vi "F Dwf Analog Impedance Amplitude Get.vi"(8 "error in (no error)":errorcluster, 10 "pvolts":dbl, 11 "hdwf":i32) -> (0 "error out":errorcluster, 2 "pvolts out":dbl, 3 "function return":i32)   [LabVIEW 2019, in "Olasdwf.lvlib"]
doc: "DWFAPI int FDwfAnalogImpedanceAmplitudeGet(HDWF hdwf, double *pvolts);"
uses:
  Olasdwf.lvlib
  Windows/System32/dwf.dll
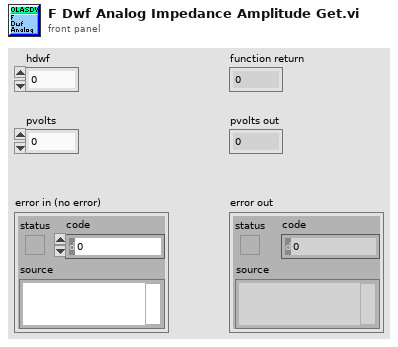
[diagram p1: front panel]
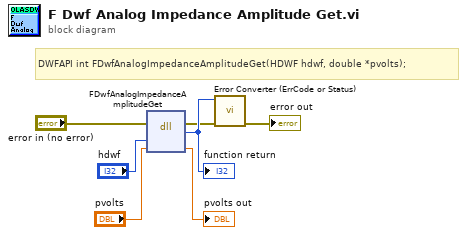
[diagram p0: block diagram]
diagram:
  # "DWFAPI int FDwfAnalogImpedanceAmplitudeGet(HDWF hdwf, double *pvolts);"
  n1 = dll-call lib="C:/Windows/System32/dwf.*" fn="FDwfAnalogImpedanceAmplitudeGet"(error in="error in (no error)", "hdwf"="hdwf", "pvolts"="pvolts") -> (error out=w2:errorcluster, w7:i32, "pvolts"=→"pvolts out":dbl)  [unwired: 3 in, 1 out]
  "function return" <- w7
  n2 = call "Error Converter (ErrCode or Status).vi"("error in (no error)"=w2, "error code"=w7) -> ("error out"=→"error out":errorcluster)  [unwired: 9 in]
